vi "Configure UVP State and Level.vi"(6 "UVP Warm(S)":dbl min=0.0 max=10.0, 7 "State":bool, 8 "error in":errorcluster, 9 "UVP Delay(S)":dbl min=0.0 max=10.0, 10 "UVP Level(V)":dbl min=0.0 max=610.0, 11 "VISA resource name":refnum<visa-resource-name>) -> (0 "error out":errorcluster, 3 "VISA resource name out":refnum<visa-resource-name>)   [LabVIEW 2018, in "IT-M3100.lvlib"]
doc: "This command enables or disables the under-voltage function.\n<b>UVP Level(V)</b>\n0-610\n<b>UVP Delay(S)</b>\n0-10\n<b>UVP Warm(S)</b>\n0-30"
uses:
  IT-M3100.lvlib
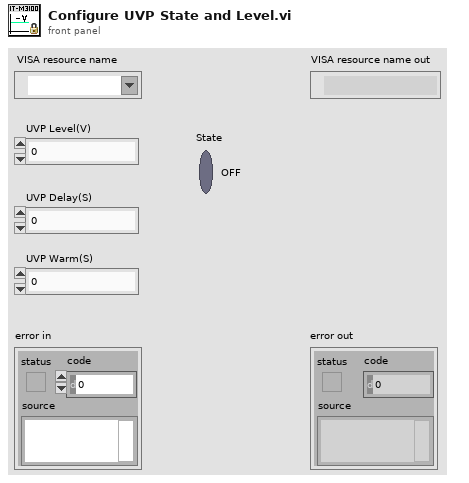
[diagram p1: front panel]
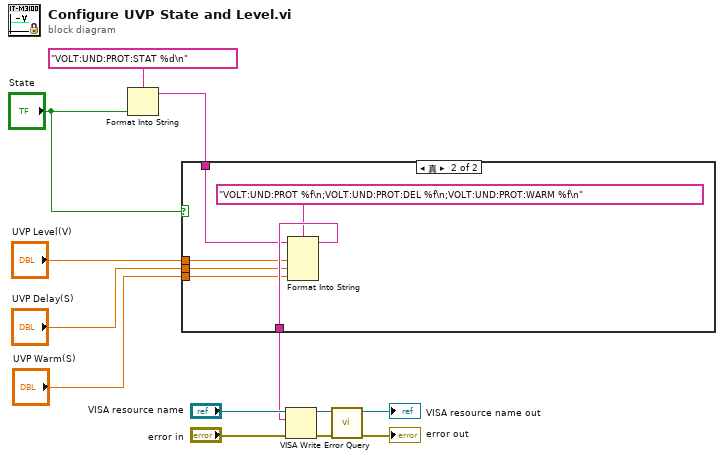
[diagram p0: block diagram]
diagram:
  n1 = Format Into String(format string="VOLT:UND:PROT:STAT %d\n", "State") -> (resulting string=w5:string)  [unwired: 2 in, 1 out]
  n2 = case shown="真" "State" {
    tunnel: w5 -> [w14 w18]
    tunnel: [w14 w20] -> w6
    tunnel: "UVP Level(V)" -> [_ w17]
    tunnel: "UVP Delay(S)" -> [_ w16]
    tunnel: "UVP Warm(S)" -> [_ w15]
    frame False {
    }
    frame True {
      n3 = Format Into String(format string="VOLT:UND:PROT %f\n;VOLT:UND:PROT:DEL %f\n;VOLT:UND:PROT:WARM %f\n", initial string=w18, w17, w16, w15) -> (resulting string=w20:string)  [unwired: 1 in, 1 out]
    }
  }
  n4 = VISA Write(VISA resource name="VISA resource name", write buffer=w6, error in (no error)="error in") -> (VISA resource name out=w10:refnum<visa-resource-name>, error out=w11:errorcluster)  [unwired: 1 out]
  n5 = call "Error Query.vi"("error in"=w11, "VISA resource name"=w10) -> ("error out"=→"error out":errorcluster, "VISA resource name out"=→"VISA resource name out":refnum<visa-resource-name>)  [unwired: 6 in, 2 out]
